vi "强制类型转换DBL to I64.vi"() -> ()   [LabVIEW 2023]
doc: "本VI是为《我和LabVIEW》一书编写的示例。\n关于本书的介绍请参考网页：\nhttp://ruanqizhen.spaces.live.com/blog/cns!5852D4F797C53FB6!4310.entry"
panel:
  out "64位整型":i64
  out "I64数据":i64 format="%.0b"
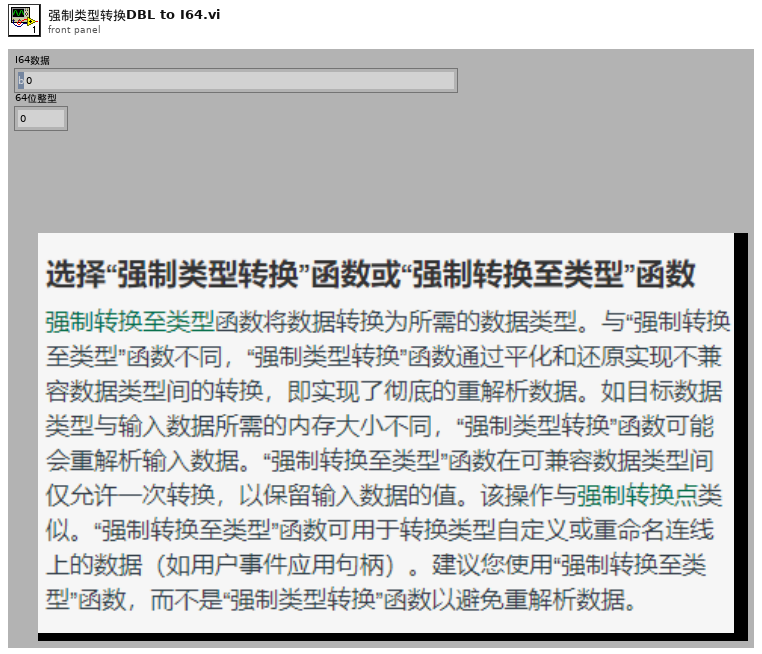
[diagram p1: front panel]
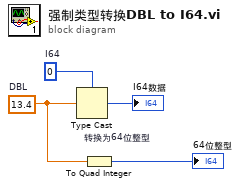
[diagram p0: block diagram]
diagram:
  w4 = i64 0  # I64
  w1 = 13.4  # DBL
  n1 = Type Cast ("强制类型转换")(type=w4, x=w1) -> (*(type *) &x=→"I64数据":i64)
  n2 = To Quad Integer "转换为64位整型"(1:w1) -> (0:→"64位整型":i64)
